vi "P cube1--front Sw.vi"(1 "P Cube1--front sw":T4, 3 "Command Info In":T1, 4 "Switch":string) -> (10 "Command Info Out":T1)   [LabVIEW 2017]
uses:
  Block Clusters/P cube1--front Sw.ctl
  <vilib>/Rock Robotics/WPI/Framework/Command Status Info.ctl
  <vilib>/Rock Robotics/WPI/Framework/Completion Status.ctl
  <vilib>/Rock Robotics/WPI/Framework/Completion Notifier.ctl
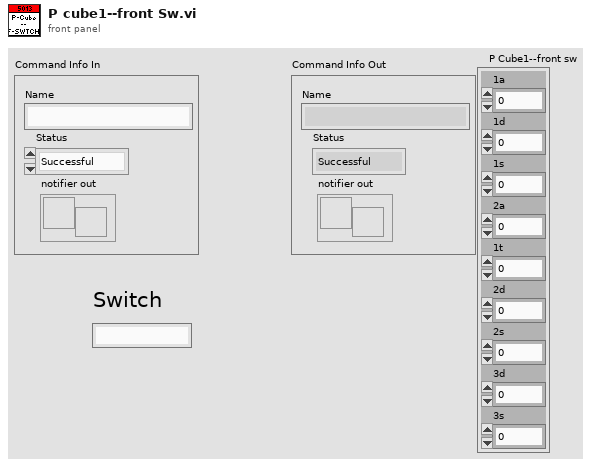
[diagram p1: front panel]
types:
  T1 = typedef "Command Status Info.ctl" = cluster{"Name":string, "Status":T2, "notifier out":T3}
  T2 = typedef "Completion Status.ctl" = enum16{"Successful", "Aborted", "Incomplete"}
  T3 = typedef "Completion Notifier.ctl" = refnum<notifier>
  T4 = typedef "P cube1--front Sw.ctl" = cluster{"1a":dbl, "1d":dbl, "1s":dbl, "2a":dbl, "1t":dbl, "2d":dbl, "2s":dbl, "3d":dbl, "3s":dbl}
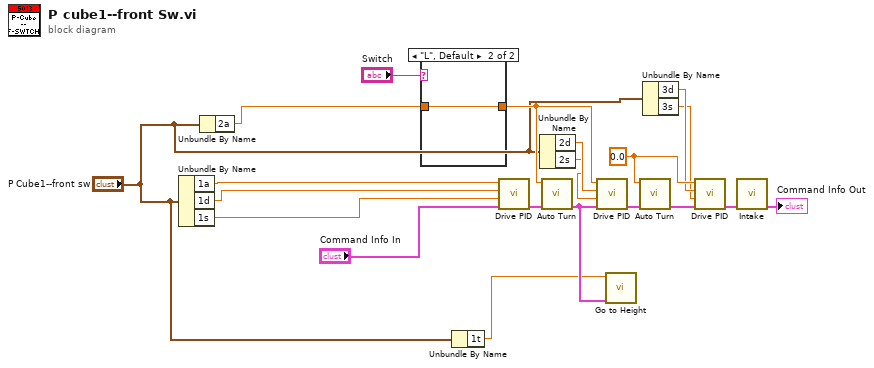
[diagram p0: block diagram]
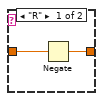
[diagram p2: hidden frame]
diagram:
  w17 = 0.0 ("Target Angle")
  n1 = Unbundle By Name("P Cube1--front sw") -> ("1a"=w14:dbl, "1d"=w13:dbl, "1s"=w12:dbl)
  n2 = Unbundle By Name("P Cube1--front sw") -> ("2a"=w10:dbl)
  n3 = case shown="\"L\", Default" "Switch" {
    tunnel: [w22 w23] -> w15
    tunnel: w10 -> [w21 w23]
    frame "R" {
      n4 = Negate(x=w21) -> (-x=w22:dbl)
    }
    frame "L", Default {
    }
  }
  n5 = Unbundle By Name("P Cube1--front sw") -> ("1t"=w3:dbl)
  n6 = call "Drive PID.vi"("Command Info In"="Command Info In", "Speed"=w12, "Distance"=w13, "Target Angle"=w14) -> ("Command Info Out"=w20:T1)  [unwired: 7 in]
  n7 = Unbundle By Name("P Cube1--front sw") -> ("2d"=w9:dbl, "2s"=w8:dbl)
  n8 = call "Auto Turn.vi"("Command Info In"=w20, "Target Angle"=w15) -> ("Command Info Out"=w19:T1)  [unwired: 9 in]
  n9 = call "Drive PID.vi"("Command Info In"=w19, "Speed"=w8, "Distance"=w9, "Target Angle"=w15) -> ("Command Info Out"=w18:T1)  [unwired: 7 in]
  n10 = call "Go to Height.vi"("Command Info In"=w19, "Target Height (in)"=w3) -> ()  [unwired: 9 in, 1 out]
  n11 = call "Auto Turn.vi"("Command Info In"=w18, "Target Angle"=w17) -> ("Command Info Out"=w2:T1)  [unwired: 9 in]
  n12 = Unbundle By Name("P Cube1--front sw") -> ("3d"=w7:dbl, "3s"=w6:dbl)
  n13 = call "Drive PID.vi"("Command Info In"=w2, "Speed"=w6, "Distance"=w7, "Target Angle"=w17) -> ("Command Info Out"=w1:T1)  [unwired: 7 in]
  n14 = call "Intake.vi"("Command Info In"=w1) -> ("Command Info Out"=→"Command Info Out":T1)  [unwired: 10 in]
